vi "frequency_sweep_0.vi"() -> ()   [LabVIEW 2016]
uses:
  <instrlib>/niVNA/niVNA.llb/niVNA Configure Frequency Start Stop.vi
  <instrlib>/niVNA/niVNA.llb/niVNA Fetch Sweep Measurement (DBL).vi
panel:
  out "SpectrumGraph":cluster{"Numeric":dbl, "real":dbl}[](graph)
  out "Error Out":errorcluster
  in  "Value":i32(ring) items=["Im", "Re", "Abs"]
  in  "Stop button":bool
  in  "S-parameter":i32(ring) caption="Measurement" items=["S11", "S21"]
  in  "Format":i32(ring) items=["Log Magnitude (dB)", "Lin Magnitude"]
  in  "Output Power":dbl=5.0
  in  "Number of Points":i32=201 min=1 max=3201
  in  "Stop Frequency":dbl=6000000000.0 min=10000000.0 max=6000000000.0 format="%#_6e"
  in  "Start Frequency":dbl=10000000.0 min=10000000.0 max=6000000000.0 format="%#_6e"
  in  "Resource Name In":refnum<k15>="PXI1Slot2"
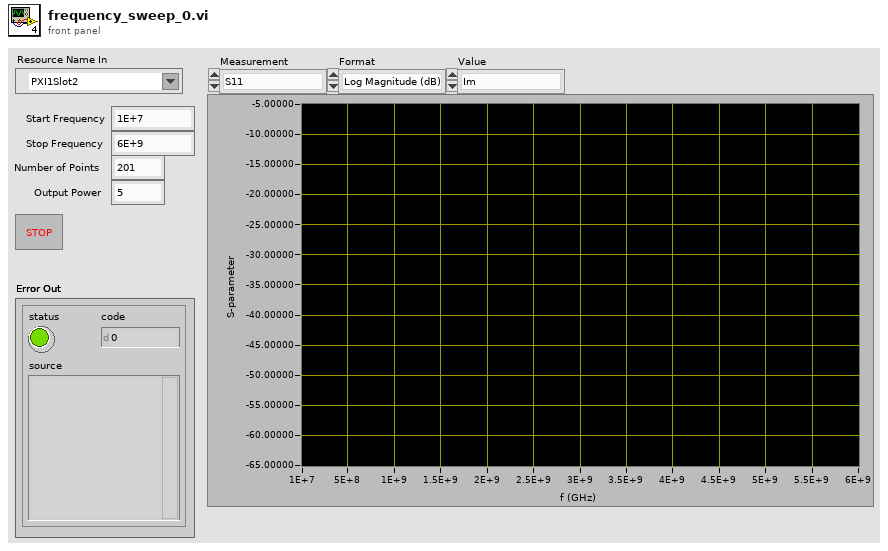
[diagram p1: front panel]
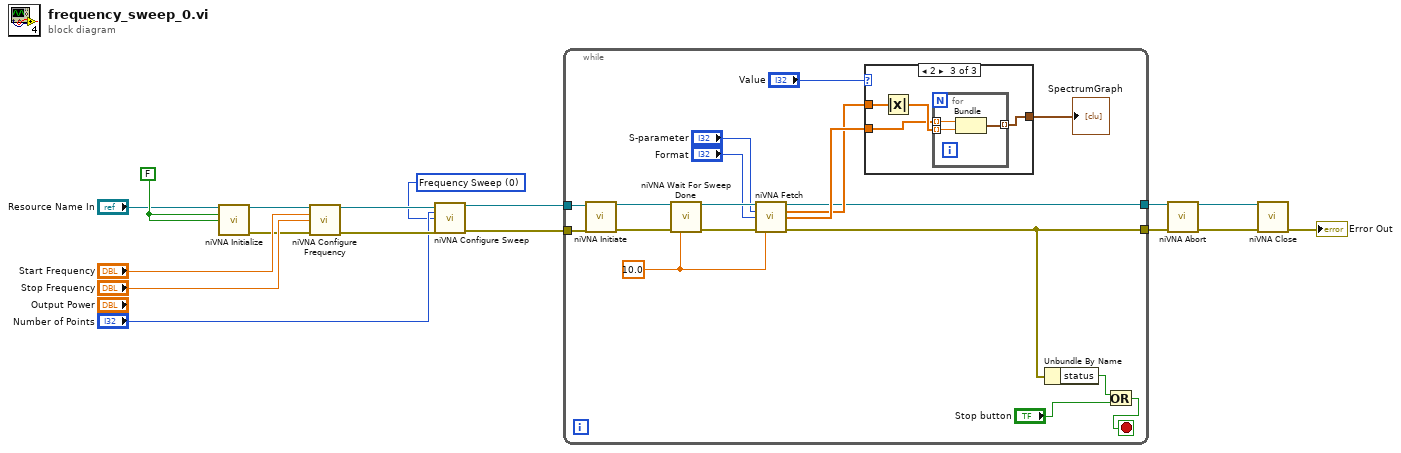
[diagram p0: block diagram]
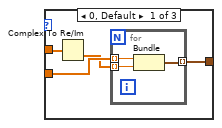
[diagram p2: hidden frame]
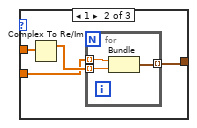
[diagram p3: hidden frame]
diagram:
  w8 = 0 items=["Frequency Sweep", "Power Sweep"] ("sweep mode")
  w17 = FALSE ("id query")
  n1 = call <instrlib>:"niVNA Initialize.vi"("resource name"="Resource Name In", "id query"=w17, "reset"=w17) -> ("instrument handle"=w12:refnum<k15>, "error out"=w13:errorcluster)  [unwired: 11 in]
  n2 = call-poly <instrlib>:"niVNA Configure Frequency.vi"("instrument handle"=w12, "start frequency"="Start Frequency", "stop frequency"="Stop Frequency", "error in"=w13) -> ("instrument handle out"=w11:refnum<k15>, "error out"=w10:errorcluster)  [unwired: 10 in]
  n3 = call <instrlib>:"niVNA Configure Sweep.vi"("instrument handle"=w11, "number of points"="Number of Points", "sweep mode"=w8, "error in"=w10) -> ("instrument handle out"=w7:refnum<k15>, "error out"=w6:errorcluster)  [unwired: 10 in]
  n4 = while {
    tunnel: w7 -> [w35]
    tunnel: w6 -> [w34]
    tunnel: [w23] -> w5
    tunnel: [w21] -> w4
    stop <- w18 stop-if-true
    w27 = 10.0 ("timeout")
    n5 = call <instrlib>:"niVNA Initiate.vi"("instrument handle"=w35, "error in"=w34) -> ("instrument handle out"=w33:refnum<k15>, "error out"=w32:errorcluster)  [unwired: 12 in]
    n6 = call <instrlib>:"niVNA Wait For Sweep Done.vi"("instrument handle"=w33, "error in"=w32, "timeout"=w27) -> ("instrument handle out"=w31:refnum<k15>, "error out"=w28:errorcluster)  [unwired: 11 in]
    n7 = call-poly <instrlib>:"niVNA Fetch.vi"("instrument handle"=w31, "measurement"="S-parameter", "format"="Format", "error in"=w28, "timeout"=w27) -> ("instrument handle out"=w23:refnum<k15>, "data"=w24:dbl[], "scale points"=w25:dbl[], "error out"=w21:errorcluster)  [unwired: 7 in]
    n8 = case shown="2" "Value" {
      tunnel: w25 -> [w39 w44 w51]
      tunnel: w24 -> [w38 w46 w53]
      tunnel: [w36 w43 w50] -> w22
      frame 0, Default {
        n9 = Complex To Re/Im(x + iy=w38) -> (y=w37:dbl[])  [unwired: 1 out]
        n10 = for {
          tunnel: w39 -> [w42] mode=indexing
          tunnel: [w41] -> w36 mode=indexing
          tunnel: w37 -> [w40] mode=indexing
          n11 = Bundle("Numeric"=w42, "Numeric"=w40) -> (w41:cluster{"Numeric":dbl, "Numeric":dbl})  [unwired: 1 in]
        }
      }
      frame 1 {
        n12 = Complex To Re/Im(x + iy=w46) -> (x=w45:dbl[])  [unwired: 1 out]
        n13 = for {
          tunnel: [w49] -> w43 mode=indexing
          tunnel: w45 -> [w48] mode=indexing
          tunnel: w44 -> [w47] mode=indexing
          n14 = Bundle("Numeric"=w47, "Numeric"=w48) -> (w49:cluster{"Numeric":dbl, "Numeric":dbl})  [unwired: 1 in]
        }
      }
      frame 2 {
        n15 = Absolute Value(x=w53) -> (abs(x)=w52:dbl[])
        n16 = for {
          tunnel: w51 -> [w56] mode=indexing
          tunnel: [w55] -> w50 mode=indexing
          tunnel: w52 -> [w54] mode=indexing
          n17 = Bundle("Numeric"=w56, "Numeric"=w54) -> (w55:cluster{"Numeric":dbl, "Numeric":dbl})  [unwired: 1 in]
        }
      }
    }
    "SpectrumGraph" <- w22
    n18 = Unbundle By Name(w21) -> ("status"=w20:bool)
    n19 = Or(x=w20, y="Stop button") -> (x .or. y?=w18:bool)
  }
  n20 = call <instrlib>:"niVNA Abort.vi"("instrument handle"=w5, "error in"=w4) -> ("instrument handle out"=w1:refnum<k15>, "error out"=w3:errorcluster)  [unwired: 12 in]
  n21 = call <instrlib>:"niVNA Close.vi"("instrument handle"=w1, "error in"=w3) -> ("error out"=→"Error Out":errorcluster)  [unwired: 13 in]
